vi "RaiseWindow.vi"(8 "No Error":errorcluster, 11 "Window [SDL_Window *]":i64) -> (0 "Error Out":errorcluster)   [LabVIEW 2024, in "SDL3.lvlib" / "Video.lvlib"]
doc: "<B>Summary</B>\nRequest that a window be raised above other windows and gain the input focus.\n\n<B>Remarks</B>\nThe result of this request is subject to desktop window manager policy, particularly if raising the requested window would result in stealing focus from another application. If the window is successfully raised and gains input focus, an <B>SDL_EVENT_WINDOW_FOCUS_GAINED</B> event will be emitted, and the window will have the <B>SDL_WINDOW_INPUT_FOCUS</B> flag set."
uses:
  Video.lvlib
  Error/Error.lvlib
  Lib/SDL3-32.dll
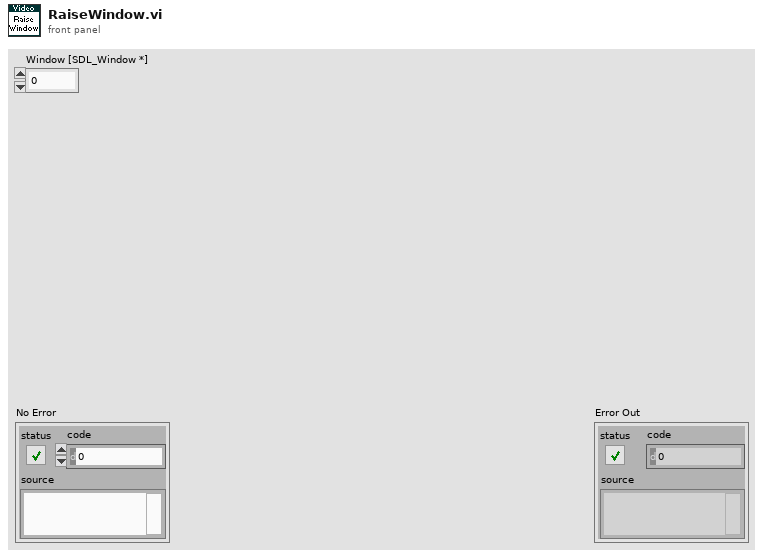
[diagram p1: front panel]
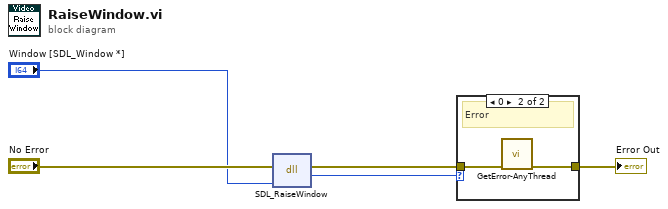
[diagram p0: block diagram]
diagram:
  n1 = dll-call lib="C:/Users/Thomas/Documents/Projects/LV-SDL3/Lib/SDL3-*.*" fn="SDL_RaiseWindow"(error in="No Error", "window"="Window [SDL_Window *]") -> (error out=w3:errorcluster, "return type"=w1:i32)  [unwired: 3 in, 1 out]
  n2 = case shown="0" w1 {
    tunnel: w3 -> [w6 w8]
    tunnel: [w6 w7] -> w2
    frame Default {
      # "Ok"
    }
    frame 0 {
      # "Error"
      n3 = call "GetError-AnyThread.vi"("No Error"=w8) -> ("Error Out"=w7:errorcluster)  [unwired: 10 in]
    }
  }
  "Error Out" <- w2
